vi "uint32 to Hex vg.vi"(11 "number":dbl) -> (1 "Hex string":string, 2 "[31:16]":string, 3 "[15:0]":string)   [LabVIEW 2020]
panel:
  # "RE-ENTRANT"
  # "SUBROUTINE"
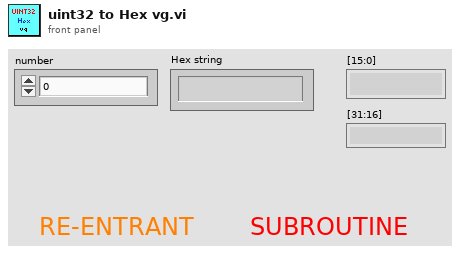
[diagram p1: front panel]
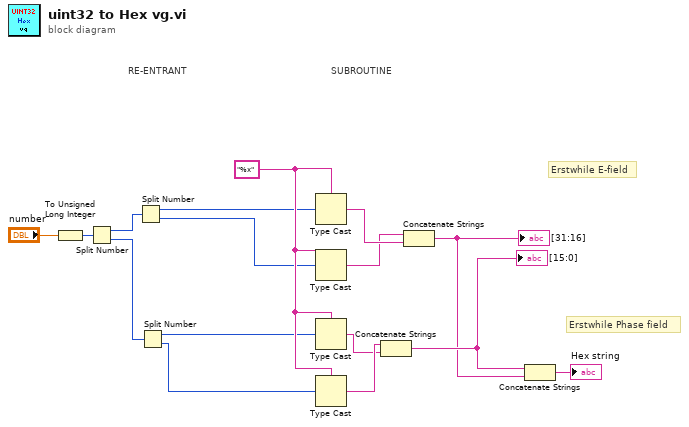
[diagram p0: block diagram]
diagram:
  w12 = "%x" ("type")
  # "Erstwhile Phase field"
  # "Erstwhile E-field"
  # "SUBROUTINE"
  # "RE-ENTRANT"
  n1 = To Unsigned Long Integer(number="number") -> (unsigned 32bit integer=w14:u32)
  n2 = Split Number(x=w14) -> (hi(x)=w15:u16, lo(x)=w16:u16)
  n3 = Split Number(x=w15) -> (hi(x)=w9:u8, lo(x)=w10:u8)
  n4 = Split Number(x=w16) -> (hi(x)=w11:u8, lo(x)=w4:u8)
  n5 = Type Cast(type=w12, x=w9) -> (*(type *) &x=w6:string)
  n6 = Type Cast(type=w12, x=w10) -> (*(type *) &x=w5:string)
  n7 = Type Cast(type=w12, x=w11) -> (*(type *) &x=w7:string)
  n8 = Type Cast(type=w12, x=w4) -> (*(type *) &x=w8:string)
  n9 = Concatenate Strings(w8, w7) -> (w2:string)
  "[15:0]" <- w2
  n10 = Concatenate Strings(w5, w6) -> (w1:string)
  "[31:16]" <- w1
  n11 = Concatenate Strings(w2, w1) -> (→"Hex string":string)
